vi "decodeDataIdentity.vi"(5 "dataIdentityCode":string) -> (2 "dataIdentityText":string)   [LabVIEW 2010]
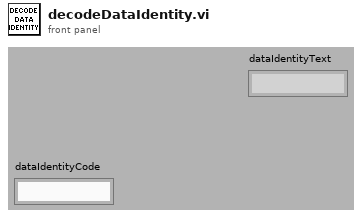
[diagram p1: front panel]
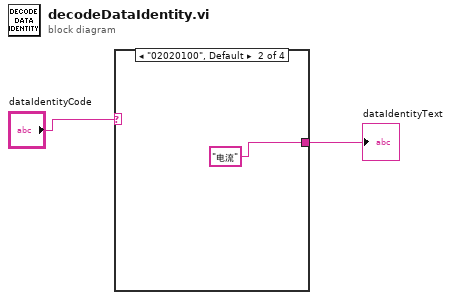
[diagram p0: block diagram]
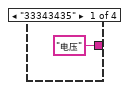
[diagram p2: hidden frame]
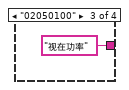
[diagram p3: hidden frame]
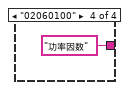
[diagram p4: hidden frame]
diagram:
  n1 = case shown="\"02020100\", Default" "dataIdentityCode" {
    tunnel: ["电压" "电流" "视在功率" "功率因数"] -> w1
    frame "33343435" {
    }
    frame "02020100", Default {
    }
    frame "02050100" {
    }
    frame "02060100" {
    }
  }
  "dataIdentityText" <- w1
